vi "Wait on BRF.vi"(8 "Error In":errorcluster, 10 "Binary Flag State":T1) -> (0 "Error Out":errorcluster)   [LabVIEW 2012]
doc: "This sub-VI waits on a flag from the Arduino (board ready flag or BRF) indicating that it is OK to move on\nto the next step."
uses:
  Controls/binary_states_enum.ctl
  <vilib>/DAQmx/read.llb/DAQmx Read (Digital Bool 1Line 1Point).vi
  <vilib>/DAQmx/miscellaneous.llb/DAQmx Fill In Error Info.vi
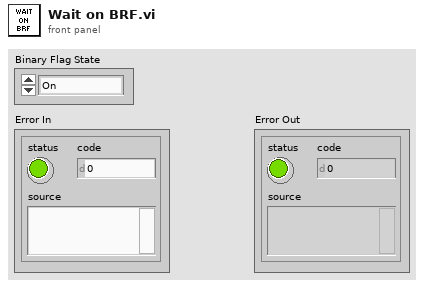
[diagram p1: front panel]
types:
  T1 = typedef "binary_states_enum.ctl" = enum16{"On", "Off"}
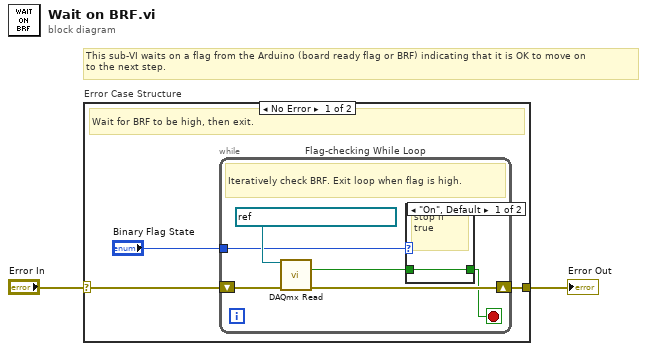
[diagram p0: block diagram]
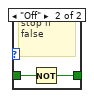
[diagram p2: hidden frame]
diagram:
  # "This sub-VI waits on a flag from the Arduino (board ready flag or BRF) indicating that it is OK to move on\nto the next step."
  n1 = case "Error Case Structure" shown="No Error" "Error In" {
    selector: "Error In" -> [w5 w15]
    tunnel: [w4 w15] -> w1
    frame No Error {
      # "Wait for BRF to be high, then exit."
      n2 = while "Flag-checking While Loop" {
        shift-right: [w10] -> w4
        shift-left: w5 -> [w11]
        tunnel: "Binary Flag State" -> [w6]
        stop <- w7 stop-if-true
        # "Iteratively check BRF. Exit loop when flag is high."
        n3 = call-poly <vilib>:"DAQmx Read.vi"("task/channels in"=refnum<k21> "BoardReadyFlag_S3P00L4", "error in"=w11) -> ("data"=w8:bool, "error out"=w10:errorcluster)  [unwired: 11 in, 1 out]
        n4 = case shown="\"On\", Default" w6 {
          tunnel: w8 -> [w12 w14]
          tunnel: [w12 w13] -> w7
          frame "On", Default {
            # "stop if\ntrue"
          }
          frame "Off" {
            # "stop if\nfalse"
            n5 = Not(x=w14) -> (.not. x?=w13:bool)
          }
        }
      }
    }
    frame Error {
      # "Pass through and exit."
    }
  }
  "Error Out" <- w1
